vi "Write Path.vi"(8 "error in (no error)":errorcluster, 10 "Path":path, 11 "File Session in":refnum<class "File Session.lvclass">=refnum) -> (0 "error out":errorcluster, 3 "File Session out":refnum<class "File Session.lvclass">)   [LabVIEW 2016, in "File Session.lvclass"]
uses:
  File Session.lvclass
  File Session.lvclass/File Session.ctl
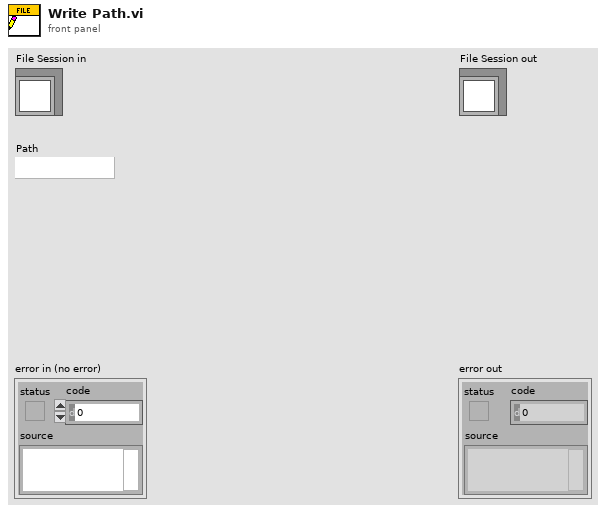
[diagram p1: front panel]
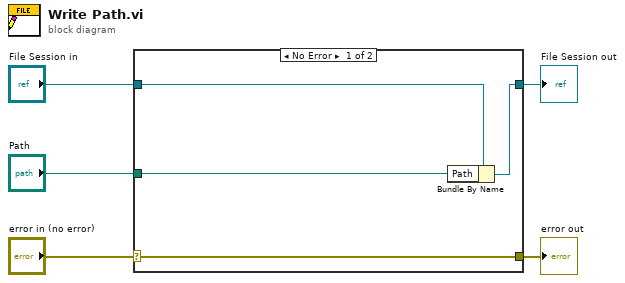
[diagram p0: block diagram]
diagram:
  n1 = case shown="No Error" "error in (no error)" {
    selector: "error in (no error)" -> [w9 w10]
    tunnel: [w9 w10] -> w4
    tunnel: [w7 w11] -> w2
    tunnel: "File Session in" -> [w8 w11]
    tunnel: "Path" -> [w6 _]
    frame No Error {
      n2 = Bundle By Name(cluster=w8, "Path"=w6) -> (w7:refnum<class "File Session.lvclass">)
    }
    frame Error {
    }
  }
  "error out" <- w4
  "File Session out" <- w2
